vi "Stanford Research SIM 921 Curve Manager.vi"(11 "VISA session":refnum<visa-resource-name>) -> ()   [LabVIEW 2020]
doc: "VI to manage calibration curves in Lakeshore model 370 AC resistance Bridge. It will upload, download and display or delete curves. It will always delete a curve before uploading so the input setup may have to be reset after an upload.\nScott Hannahs, <sth@magnet.fsu.edu> NHMFL-FSU, May 2003"
panel:
  in  "Done2":bool
  out "XY Graph":cluster{dbl[], dbl[]}(graph)
  out "Curve #":i32[](array[numeric])
  in  "Active":T1(radio)
  in  "SIM Slot #":T2(radio)
  in  "stop":bool
  in  "Replace":bool[](array[boolean])=[FALSE, FALSE, FALSE, FALSE, FALSE, FALSE, FALSE, FALSE, FALSE, FALSE, FALSE, FALSE, FALSE, FALSE, FALSE, FALSE, FALSE, FALSE, FALSE, FALSE]
  in  "View":bool[](array[boolean])=[FALSE, FALSE, FALSE, FALSE, FALSE, FALSE, FALSE, FALSE, FALSE, FALSE, FALSE, FALSE, FALSE, FALSE, FALSE, FALSE, FALSE, FALSE, FALSE, FALSE]
  in  "Delete":bool[](array[boolean])=[FALSE, FALSE, FALSE, FALSE, FALSE, FALSE, FALSE, FALSE, FALSE, FALSE, FALSE, FALSE, FALSE, FALSE, FALSE, FALSE, FALSE, FALSE, FALSE, FALSE]
  out "Thermometer List":T3(array[cluster])
  out "Model":string="LakeShore Model 370"
  out "Info":string="S/N #000000, Software Date: 20030622"
  # "Name"
  # "Serial #"
  # "Data Format"
  # "# Points"
  # "`"
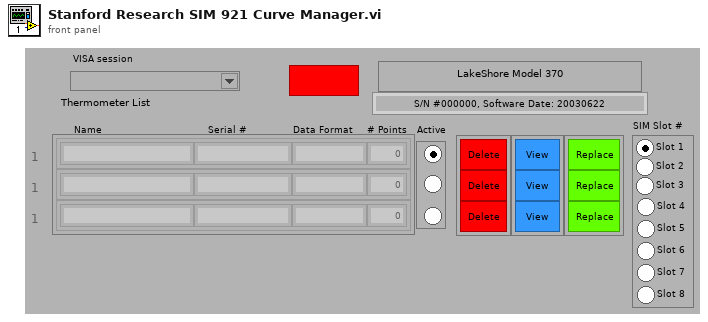
[diagram p1: front panel]
types:
  T1 = enum32{"Radio Selection 1", "Radio Selection 2", "Radio Selection 3"}
  T2 = enum32{"Slot 1", "Slot 2", "Slot 3", "Slot 4", "Slot 5", "Slot 6", "Slot 7", "Slot 8"}
  T3 = cluster{"Name":string, "Serial #":string, "String":string, "Number of Points":dbl}[]
  T4 = cluster{"Curve ID":string, "Serial Number":string, "Data Format":string, "Number of Points":u32}[]
  T5 = cluster{"Curve ID":string, "Serial Number":string, "Data Format":string, "Number of Points":u32}
  T6 = enum16{"Linear", "SemiLogT", "SemiLogR", "LogLog"}
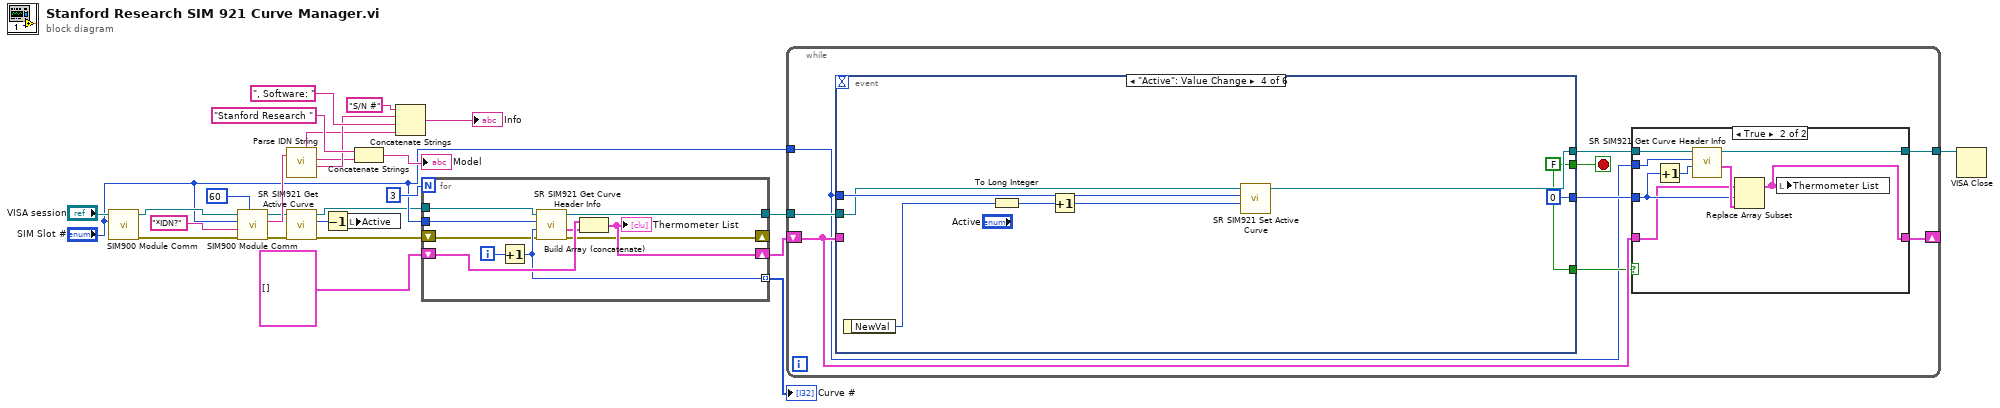
[diagram p0: block diagram]
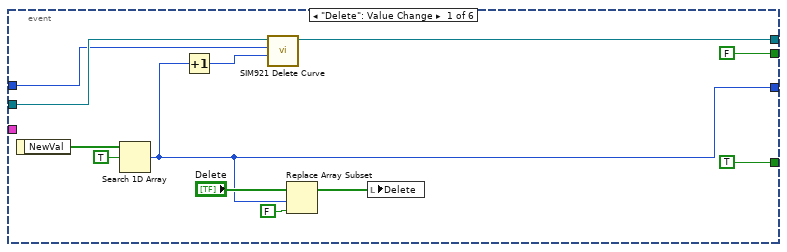
[diagram p3: hidden frame]
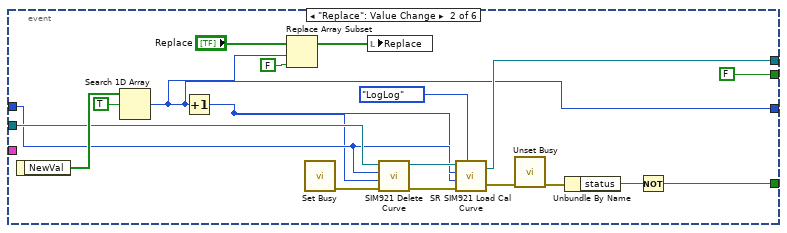
[diagram p4: hidden frame]
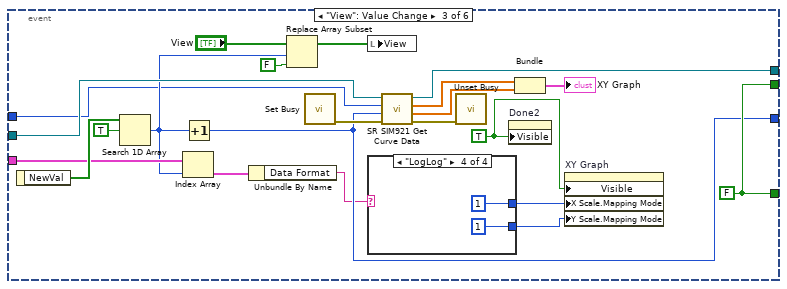
[diagram p5: hidden frame]
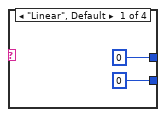
[diagram p6: hidden frame]
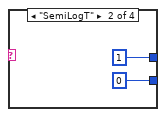
[diagram p7: hidden frame]
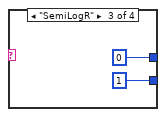
[diagram p8: hidden frame]
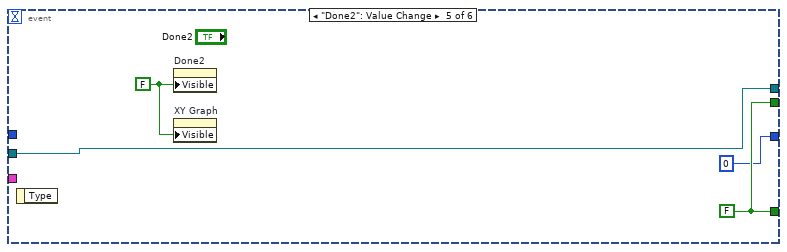
[diagram p9: hidden frame]
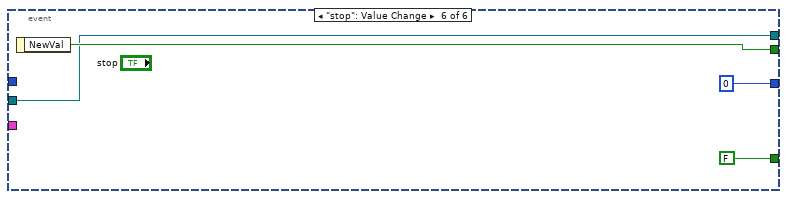
[diagram p10: hidden frame]
diagram:
  n1 = call "SIM900 Module Comm.vi"("Slot"="SIM Slot #", "VISA Resource Name"="VISA session") -> ("Error Out"=w7:errorcluster, "dup VISA Session"=w9:refnum<visa-resource-name>)  [unwired: 7 in, 1 out]
  n2 = call "SIM900 Module Comm.vi"("Wait (ms)"=u32 60, "Error In"=w7, "Query"="*IDN?" ("String to Write"), "Slot"="SIM Slot #", "VISA Resource Name"=w9) -> ("Error Out"=w6:errorcluster, "Response"=w18:string, "dup VISA Session"=w4:refnum<visa-resource-name>)  [unwired: 4 in]
  n3 = call "Parse IDN String.vi"("IDN String"=w18) -> ("Info"=w17:string, "Model"=w14:string, "Revision"=w16:string)  [unwired: 1 in, 2 out]
  n4 = call "SR SIM921 Get Active Curve.vi"("Error In"=w6, "VISA session"=w4) -> ("Error Out"=w5:errorcluster, "Curve #"=w2:i32, "dup VISA session"=w3:refnum<visa-resource-name>)  [unwired: 3 in]
  n5 = Decrement(x=w2) -> (x-1=w1:i32)
  n6 = local write "Active"(w1) -> ()
  n7 = Concatenate Strings("Stanford Research " ("string"), w14) -> (→"Model":string)
  n8 = Concatenate Strings("S/N #" ("string"), w17, ", Software: " ("string"), w16) -> (→"Info":string)
  n9 = for {
    N: 3 -> [_]
    tunnel: w3 -> [w37]
    shift-right: [w34] -> w26
    shift-left: T4 [] -> [w33]
    tunnel: [w35] -> w27
    tunnel: "SIM Slot #" -> [w32]
    tunnel: [w31] -> w13 mode=indexing
    shift-right: [w28] -> _
    shift-left: w5 -> [w29]
    i -> [w36]
    n10 = Increment(x=w36) -> (x+1=w31:i32)
    n11 = call "SR SIM921 Get Curve Header Info.vi"("Error In"=w29, "Curve #"=w31, "SIM Slot #"=w32, "VISA session"=w37) -> ("Error Out"=w28:errorcluster, "Curve Header"=w30:T5, "dup VISA session"=w35:refnum<visa-resource-name>)  [unwired: 1 in]
    n12 = Build Array (concatenate)(w33, w30) -> (w34:T4)
    "Thermometer List" <- w34
  }
  "Curve #" <- w13
  n13 = while {
    tunnel: w27 -> [w46]
    shift-right: [w41] -> _
    shift-left: w26 -> [w42]
    tunnel: [w40] -> w11
    tunnel: "SIM Slot #" -> [w38]
    stop <- w43 stop-if-true
    n14 = event shown="[3] \"Active\": Value Change" {
      selector: _ -> [_ _ _ _ _ _]
      dyn-events: _ -> [_ _ _ _ _ _]
      timeout: _ -> [_ _ _ _ _ _]
      tunnel: w46 -> [w66 w75 w107 w123 w126 w131]
      tunnel: [TRUE ("NewVal") w77 w104 w121 w128 FALSE] -> w39
      tunnel: [w59 w69 w92 0 ("index of element") 0 ("index of element") 0 ("index of element")] -> w45
      tunnel: [w65 w85 w106 w122 w126 w131] -> w44
      tunnel: [FALSE ("NewVal") FALSE ("NewVal") w104 w121 w128 w133] -> w43
      tunnel: w42 -> [_ _ w105 _ _ _]
      tunnel: w38 -> [w58 w72 w90 w124 _ _]
      event "Delete": Value Change {
        n15 = event-data() -> ("NewVal"=w68:bool[])  [unwired: 1 in]
        n16 = Search 1D Array(1D array=w68, element=TRUE) -> (index of element=w59:i32)  [unwired: 1 in]
        n17 = Increment(x=w59) -> (x+1=w57:i32)
        n18 = call "SIM921 Delete Curve.vi"("Curve #"=w57, "Slot"=w58, "VISA resource name"=w66) -> ("VISA resource name"=w65:refnum<visa-resource-name>)  [unwired: 7 in, 1 out]
        n19 = Replace Array Subset(array="Delete", new element=FALSE ("new element/subarray"), index=w59) -> (w61:bool[])
        n20 = local write "Delete"(w61) -> ()
      }
      event "Replace": Value Change {
        n21 = event-data() -> ("NewVal"=w86:bool[])  [unwired: 1 in]
        n22 = Search 1D Array(1D array=w86, element=TRUE) -> (index of element=w69:i32)  [unwired: 1 in]
        n23 = Increment(x=w69) -> (x+1=w71:i32)
        n24 = Replace Array Subset(array="Replace", new element=FALSE ("new element/subarray"), index=w69) -> (w82:bool[])
        n25 = call <vilib>:"Set Busy.vi"() -> ("error out"=w74:errorcluster)  [unwired: 10 in, 1 out]
        n26 = local write "Replace"(w82) -> ()
        n27 = call "SIM921 Delete Curve.vi"("Error In"=w74, "Curve #"=w71, "Slot"=w72, "VISA resource name"=w75) -> ("Error Out"=w73:errorcluster, "VISA resource name"=w76:refnum<visa-resource-name>)  [unwired: 6 in]
        n28 = call "SR SIM921 Load Cal Curve.vi"("VISA resource name"=w76, "Slot"=w72, "Curve #"=w71, "Error In"=w73, "Curve Data Format"=T6."LogLog") -> ("dup VISA resource name"=w85:refnum<visa-resource-name>, "Error Out"=w80:errorcluster)
        n29 = call <vilib>:"Unset Busy.vi"("error in (no error)"=w80) -> ("error out"=w79:errorcluster)  [unwired: 10 in]
        n30 = Unbundle By Name(w79) -> ("status"=w78:bool)
        n31 = Not(x=w78) -> (.not. x?=w77:bool)
      }
      event "View": Value Change {
        w100 = TRUE ("Visible")
        w104 = FALSE ("NewVal")
        n32 = event-data() -> ("NewVal"=w108:bool[])  [unwired: 1 in]
        n33 = Search 1D Array(1D array=w108, element=TRUE) -> (index of element=w93:i32)  [unwired: 1 in]
        n34 = Index Array(array=w105, index=w93) -> (element=w99:T5)
        n35 = Increment(x=w93) -> (x+1=w92:i32)
        n36 = Unbundle By Name(w99) -> ("Data Format"=w89:string)
        n37 = Replace Array Subset(array="View", new element=FALSE ("new element/subarray"), index=w93) -> (w96:bool[])
        n38 = call <vilib>:"Set Busy.vi"() -> ("error out"=w95:errorcluster)  [unwired: 10 in, 1 out]
        n39 = local write "View"(w96) -> ()
        n40 = case shown="\"LogLog\"" w89 {
          tunnel: [u8 0 ("X Scale.Mapping Mode") u8 0 ("X Scale.Mapping Mode") u8 1 ("X Scale.Mapping Mode") u8 1 ("X Scale.Mapping Mode")] -> w91
          tunnel: [u8 0 ("X Scale.Mapping Mode") u8 1 ("X Scale.Mapping Mode") u8 0 ("X Scale.Mapping Mode") u8 1 ("X Scale.Mapping Mode")] -> w88
          frame "Linear", Default {
          }
          frame "SemiLogT" {
          }
          frame "SemiLogR" {
          }
          frame "LogLog" {
          }
        }
        n41 = call "SR SIM921 Get Curve Data.vi"("error in (no error)"=w95, "Curve #"=w92, "Mainframe slot"=w90, "VISA session"=w107) -> ("error out"=w94:errorcluster, "Resistance"=w103:dbl[], "Temperature"=w102:dbl[], "dup VISA session"=w106:refnum<visa-resource-name>)
        n42 = call <vilib>:"Unset Busy.vi"("error in (no error)"=w94) -> ()  [unwired: 10 in, 1 out]
        n43 = property on="Done2" class="Bool"("Visible"=w100) -> ()  [unwired: 2 in, 2 out]
        n44 = Bundle("Temperature"=w102, "Resistance"=w103) -> (→"XY Graph":cluster{"Temperature":dbl[], "Resistance":dbl[]})  [unwired: 1 in]
        n45 = property on="XY Graph" class="XYGraph (strict)"("Visible"=w100, "X Scale.Mapping Mode"=w88, "Y Scale.Mapping Mode"=w91) -> ()  [unwired: 2 in, 2 out]
      }
      event "Active": Value Change {
        w121 = FALSE ("NewVal")
        n46 = event-data() -> ("NewVal"=w125:T1)  [unwired: 1 in]
        n47 = To Long Integer(number=w125) -> (32bit integer=w118:i32)
        n48 = Increment(x=w118) -> (x+1=w119:i32)
        n49 = call "SR SIM921 Set Active Curve.vi"("Curve #"=w119, "SIM Slot #"=w124, "VISA session"=w123) -> ("dup VISA session"=w122:refnum<visa-resource-name>)  [unwired: 3 in, 1 out]
      }
      event "Done2": Value Change {
        w128 = FALSE
        w129 = FALSE ("Visible")
        n50 = event-data() -> ()  [unwired: 1 in, 1 out]
        n51 = property on="Done2" class="Bool"("Visible"=w129) -> ()  [unwired: 2 in, 2 out]
        n52 = property on="XY Graph" class="XYGraph (strict)"("Visible"=w129) -> ()  [unwired: 2 in, 2 out]
      }
      event "stop": Value Change {
        n53 = event-data() -> ("NewVal"=w133:bool)  [unwired: 1 in]
      }
    }
    n54 = case shown="True" w39 {
      tunnel: w45 -> [_ w55]
      tunnel: w44 -> [w47 w54]
      tunnel: w42 -> [w48 w53]
      tunnel: [w48 w51] -> w41
      tunnel: [w47 w52] -> w40
      tunnel: w38 -> [_ w49]
      frame False {
      }
      frame True {
        n55 = Increment(x=w55) -> (x+1=w50:i32)
        n56 = call "SR SIM921 Get Curve Header Info.vi"("Curve #"=w50, "SIM Slot #"=w49, "VISA session"=w54) -> ("Curve Header"=w56:T5, "dup VISA session"=w52:refnum<visa-resource-name>)  [unwired: 2 in, 1 out]
        n57 = Replace Array Subset(array=w53, new element=w56, index=w55) -> (w51:T4)
        n58 = local write "Thermometer List"(w51) -> ()
      }
    }
  }
  n59 = VISA Close(VISA resource name=w11) -> ()  [unwired: 1 in, 1 out]
